vi "Frame.Settings.vi"(6 "Action":enum8{"Get", "Set"}(ring), 8 "error in (no error)":errorcluster, 10 "Frame.Settings":T1={"ID"=0, "Disable Transmission"=FALSE, "Disable Transmission Ref"=18446744073709551615, "Transmit Trigger"=enum."Channel value change", "Transmit Trigger Ref"=18446744073709551615, "Start Time Offset (ms)"=0} {"Transmit Trigger Ref" format="%.0x"; "Disable Transmission Ref" format="%.0x"}, 11 "Item Ref in":T2 format="%.0x") -> (0 "error out":errorcluster, 2 "Frame.Settings":T1={"ID"=0, "Disable Transmission"=FALSE, "Disable Transmission Ref"=18446744073709551615, "Transmit Trigger"=enum."Channel value change", "Transmit Trigger Ref"=18446744073709551615, "Start Time Offset (ms)"=0} {"Transmit Trigger Ref" format="%.0x"; "Disable Transmission Ref" format="%.0x"}, 3 "Item Ref out":T2 format="%.0x")   [LabVIEW 2023, in "Protection and Counter Addon System Explorer.lvlib"]
uses:
  Protection and Counter Addon System Explorer.lvlib
  <vilib>/NI VeriStand/Custom Device API/Custom Device Item Ref.ctl
  Types/Frame Settings.ctl
  Types/Event Trigger Type.ctl
  Addon Shared/SubVIs/GUID Lookup.vi
  <vilib>/NI VeriStand/Custom Device API/Set Item Property (Dependent Node Pointer).vi
  <vilib>/NI VeriStand/Custom Device API/Set Item Property (U32).vi
  <vilib>/NI VeriStand/Custom Device API/Set Item Property (Boolean).vi
  <vilib>/NI VeriStand/Custom Device API/Get Item Property (Dependent Node Pointer).vi
  <vilib>/NI VeriStand/Custom Device API/Get Item Property (U32).vi
  <vilib>/NI VeriStand/Custom Device API/Get Item Property (Boolean).vi
  <vilib>/NI VeriStand/Custom Device API/Custom Device API.lvlib
  Addon Shared/Protection and Counter Addon Shared.lvlib
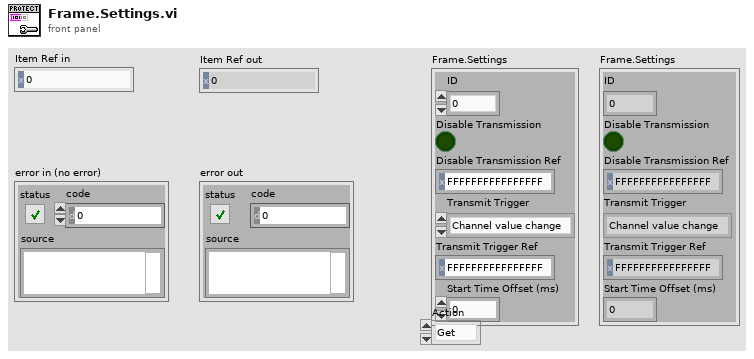
[diagram p1: front panel]
types:
  T1 = typedef "Protection and Counter Addon System Explorer.lvlib/Frame Settings.ctl" = cluster{"ID":u32, "Disable Transmission":bool, "Disable Transmission Ref":T2, "Transmit Trigger":T3, "Transmit Trigger Ref":T2, "Start Time Offset (ms)":u32}
  T2 = typedef "Custom Device API.lvlib/Custom Device Item Ref.ctl" = u64
  T3 = typedef "Protection and Counter Addon System Explorer.lvlib/Event Trigger Type.ctl" = enum16{"Channel value change", "Trigger channel (not zero)", "Channel value change or trigger channel (not zero)", "Trigger channel (any value change)", "Channel value change or trigger channel (any value change)"}
  T4 = typedef "Custom Device API.lvlib/Custom Device Item Info.ctl" = cluster{"Name":string, "Is Channel":bool, "GUID":string, "Is Waveform":bool}
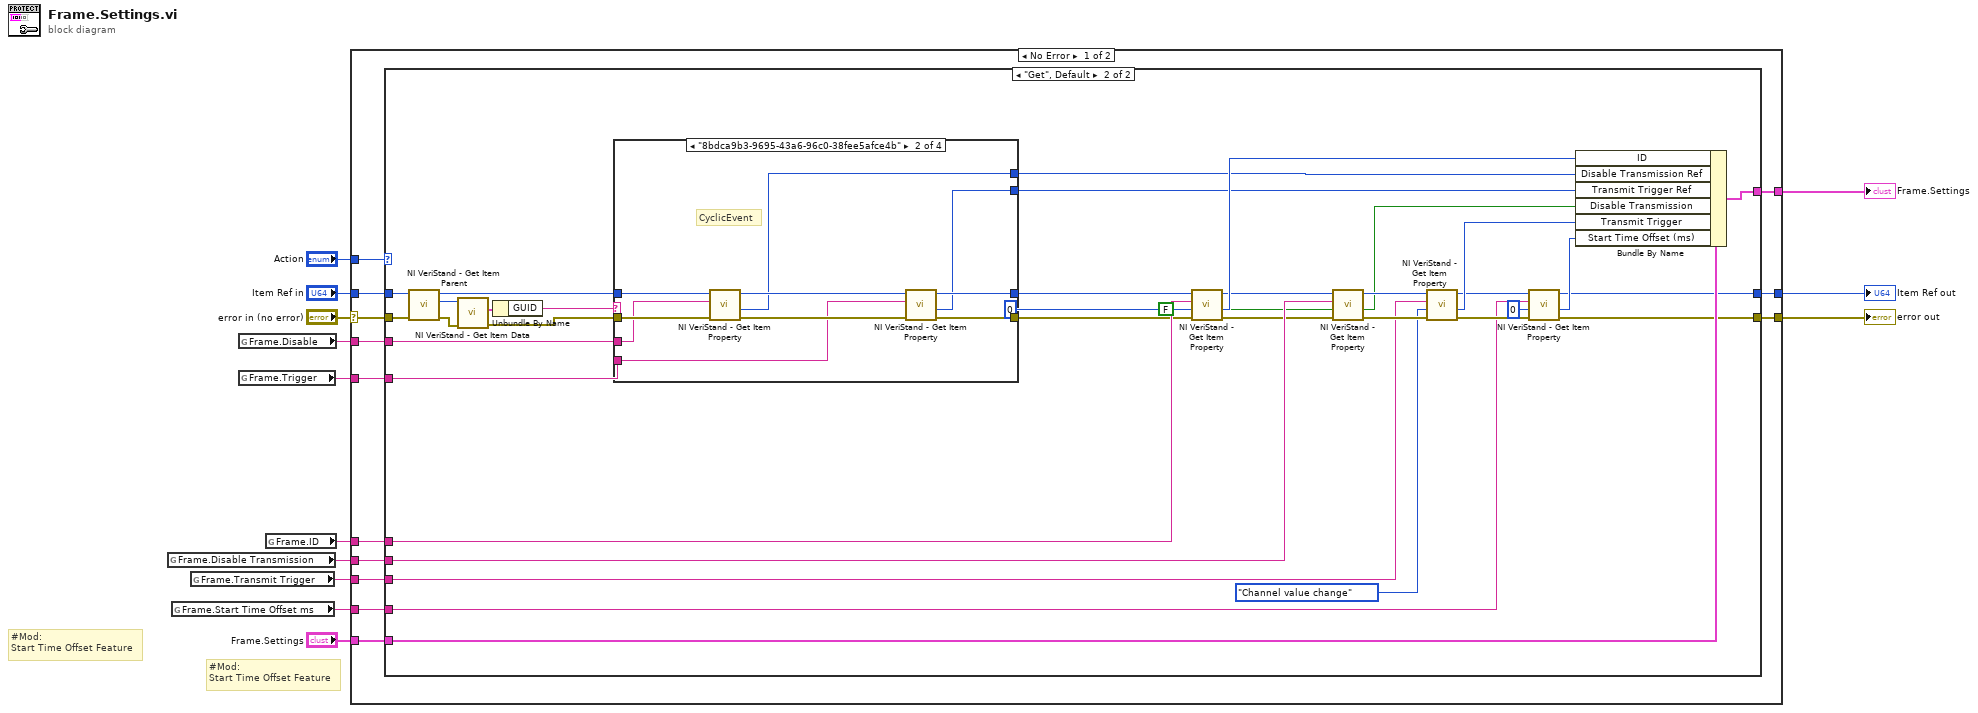
[diagram p0: block diagram]
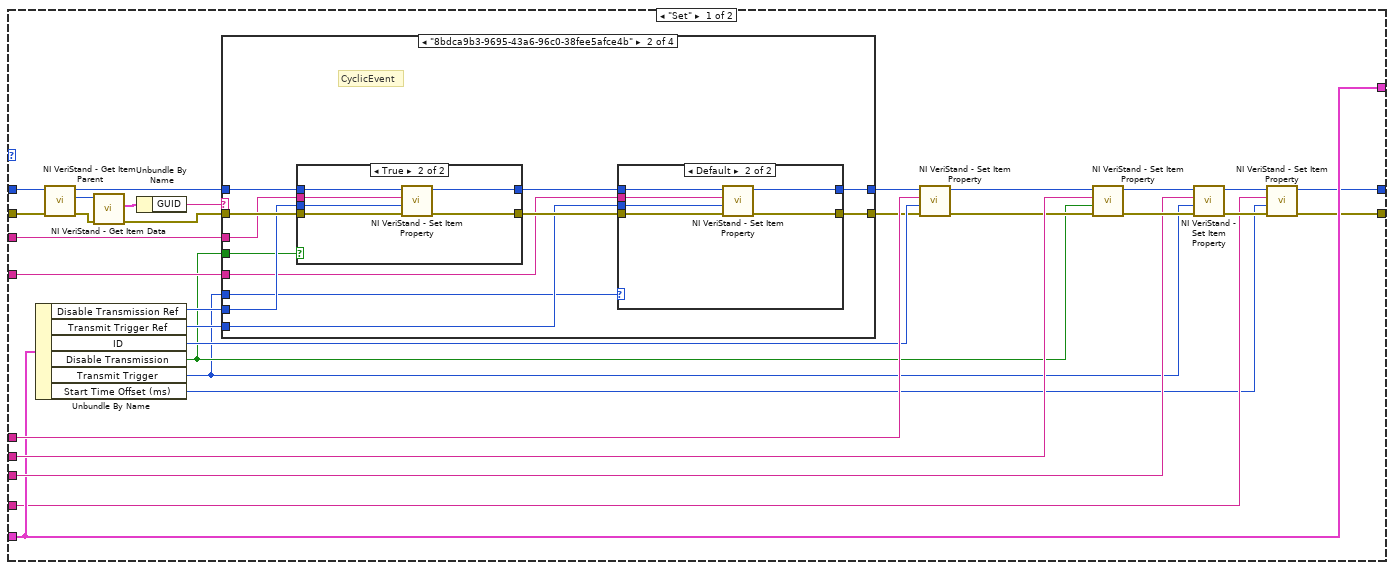
[diagram p2: hidden frame]
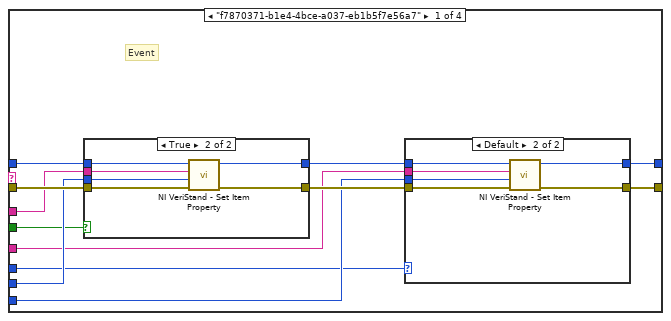
[diagram p3: hidden frame]
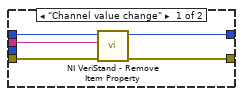
[diagram p4: hidden frame]
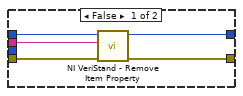
[diagram p5: hidden frame]
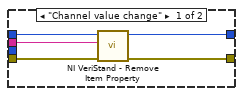
[diagram p6: hidden frame]
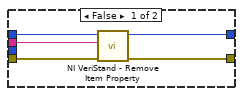
[diagram p7: hidden frame]
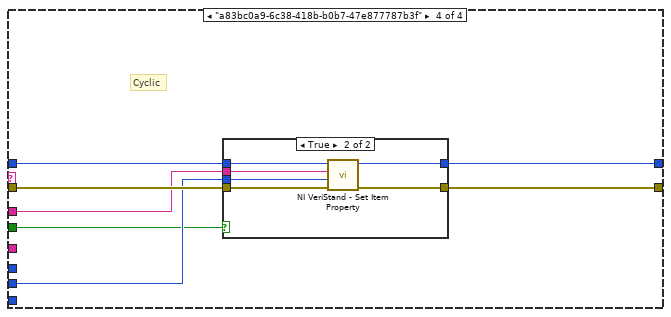
[diagram p9: hidden frame]
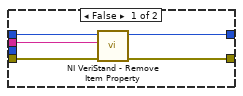
[diagram p10: hidden frame]
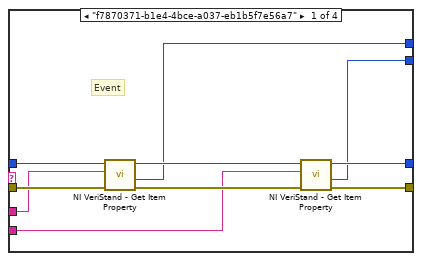
[diagram p11: hidden frame]
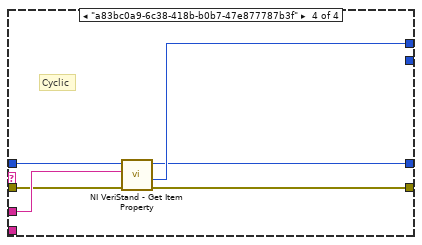
[diagram p13: hidden frame]
diagram:
  # "#Mod:\nStart Time Offset Feature"
  # "#Mod:\nStart Time Offset Feature"
  n1 = global read "GUID Lookup.vi" "Frame.Disable Transmission"() -> (w5:string)
  n2 = global read "GUID Lookup.vi" "Frame.Start Time Offset ms"() -> (w1:string)
  n3 = global read "GUID Lookup.vi" "Frame.Transmit Trigger"() -> (w6:string)
  n4 = global read "GUID Lookup.vi" "Frame.Disable"() -> (w2:string)
  n5 = global read "GUID Lookup.vi" "Frame.Trigger"() -> (w3:string)
  n6 = global read "GUID Lookup.vi" "Frame.ID"() -> (w4:string)
  n7 = case shown="No Error" "error in (no error)" {
    selector: "error in (no error)" -> [w17 w210]
    tunnel: "Item Ref in" -> [w26 w209]
    tunnel: w4 -> [w25 _]
    tunnel: w2 -> [w24 _]
    tunnel: w3 -> [w23 _]
    tunnel: [w22 w210] -> w12
    tunnel: [w21 w209] -> w11
    tunnel: [w20 _] -> w10
    tunnel: w6 -> [w19 _]
    tunnel: w5 -> [w18 _]
    tunnel: "Frame.Settings" -> [w16 _]
    tunnel: "Action" -> [w15 _]
    tunnel: w1 -> [w14 _]
    frame No Error {
      n8 = case shown="\"Get\", Default" w15 {
        tunnel: w26 -> [w45 w162]
        tunnel: w25 -> [w56 w180]
        tunnel: w24 -> [w42 w157]
        tunnel: w23 -> [w41 w156]
        tunnel: [w31 w145] -> w22
        tunnel: [w27 w146] -> w21
        tunnel: [w51 w170] -> w20
        tunnel: w19 -> [w53 w176]
        tunnel: w18 -> [w52 w175]
        tunnel: w17 -> [w44 w159]
        tunnel: w16 -> [w51 w171]
        tunnel: w14 -> [w29 w149]
        frame "Set" {
          n9 = Unbundle By Name(w51) -> ("Disable Transmission Ref"=w36:T2, "Transmit Trigger Ref"=w35:T2, "ID"=w50:u32, "Disable Transmission"=w34:bool, "Transmit Trigger"=w33:T3, "Start Time Offset (ms)"=w28:u32)
          n10 = call <vilib>:"NI VeriStand - Get Item Parent.vi"("error in (no error)"=w44, "Item Ref in"=w45) -> ("error out"=w40:errorcluster, "Parent Ref"=w47:T2, "Item Ref out"=w46:T2)  [unwired: 6 in, 1 out]
          n11 = call <vilib>:"NI VeriStand - Get Item Data.vi"("error in (no error)"=w40, "Item Ref in"=w47) -> ("error out"=w43:errorcluster, "Item Info"=w48:T4)  [unwired: 8 out]
          n12 = Unbundle By Name(w48) -> ("GUID"=w49:string)
          n13 = case shown="\"8bdca9b3-9695-43a6-96c0-38fee5afce4b\"" w49 {
            tunnel: w43 -> [w68 w102 w126 w133]
            tunnel: [w58 w92 w126 w128] -> w39
            tunnel: w42 -> [w67 w101 _ w131]
            tunnel: w41 -> [w61 w95 _ _]
            tunnel: w46 -> [w66 w100 w125 w130]
            tunnel: [w59 w93 w125 w129] -> _
            tunnel: w36 -> [w65 w99 _ w132]
            tunnel: w35 -> [w62 w96 _ _]
            tunnel: w34 -> [w64 w98 _ w127]
            tunnel: w33 -> [w57 w91 _ _]
            frame "f7870371-b1e4-4bce-a037-eb1b5f7e56a7" {
              # "Event"
              n14 = case shown="True" w64 {
                tunnel: [w80 w90] -> w60
                tunnel: [w81 w89] -> w63
                tunnel: w68 -> [w82 w88]
                tunnel: w67 -> [w83 w87]
                tunnel: w66 -> [w84 w86]
                tunnel: w65 -> [_ w85]
                frame False {
                  n15 = call <vilib>:"NI VeriStand - Remove Item Property.vi"("error in (no error)"=w82, "Property Name"=w83, "Item Ref in"=w84) -> ("error out"=w81:errorcluster, "Item Ref out"=w80:T2)  [unwired: 6 in, 1 out]
                }
                frame True {
                  n16 = call-poly <vilib>:"NI VeriStand - Set Item Property.vi"("error in (no error)"=w88, "Dependent Node Ref"=w85, "Property Name"=w87, "Item Ref in"=w86) -> ("error out"=w89:errorcluster, "Item Ref out"=w90:T2)  [unwired: 5 in, 1 out]
                }
              }
              n17 = case shown="Default" w57 {
                tunnel: [w69 w79] -> w59
                tunnel: [w70 w78] -> w58
                tunnel: w63 -> [w71 w77]
                tunnel: w61 -> [w72 w76]
                tunnel: w60 -> [w73 w75]
                tunnel: w62 -> [_ w74]
                frame "Channel value change" {
                  n18 = call <vilib>:"NI VeriStand - Remove Item Property.vi"("error in (no error)"=w71, "Property Name"=w72, "Item Ref in"=w73) -> ("error out"=w70:errorcluster, "Item Ref out"=w69:T2)  [unwired: 6 in, 1 out]
                }
                frame Default {
                  n19 = call-poly <vilib>:"NI VeriStand - Set Item Property.vi"("error in (no error)"=w77, "Dependent Node Ref"=w74, "Property Name"=w76, "Item Ref in"=w75) -> ("error out"=w78:errorcluster, "Item Ref out"=w79:T2)  [unwired: 5 in, 1 out]
                }
              }
            }
            frame "8bdca9b3-9695-43a6-96c0-38fee5afce4b" {
              # "CyclicEvent"
              n20 = case shown="True" w98 {
                tunnel: [w114 w124] -> w94
                tunnel: [w115 w123] -> w97
                tunnel: w102 -> [w116 w122]
                tunnel: w101 -> [w117 w121]
                tunnel: w100 -> [w118 w120]
                tunnel: w99 -> [_ w119]
                frame False {
                  n21 = call <vilib>:"NI VeriStand - Remove Item Property.vi"("error in (no error)"=w116, "Property Name"=w117, "Item Ref in"=w118) -> ("error out"=w115:errorcluster, "Item Ref out"=w114:T2)  [unwired: 6 in, 1 out]
                }
                frame True {
                  n22 = call-poly <vilib>:"NI VeriStand - Set Item Property.vi"("error in (no error)"=w122, "Dependent Node Ref"=w119, "Property Name"=w121, "Item Ref in"=w120) -> ("error out"=w123:errorcluster, "Item Ref out"=w124:T2)  [unwired: 5 in, 1 out]
                }
              }
              n23 = case shown="Default" w91 {
                tunnel: [w103 w113] -> w93
                tunnel: [w104 w112] -> w92
                tunnel: w97 -> [w105 w111]
                tunnel: w95 -> [w106 w110]
                tunnel: w94 -> [w107 w109]
                tunnel: w96 -> [_ w108]
                frame "Channel value change" {
                  n24 = call <vilib>:"NI VeriStand - Remove Item Property.vi"("error in (no error)"=w105, "Property Name"=w106, "Item Ref in"=w107) -> ("error out"=w104:errorcluster, "Item Ref out"=w103:T2)  [unwired: 6 in, 1 out]
                }
                frame Default {
                  n25 = call-poly <vilib>:"NI VeriStand - Set Item Property.vi"("error in (no error)"=w111, "Dependent Node Ref"=w108, "Property Name"=w110, "Item Ref in"=w109) -> ("error out"=w112:errorcluster, "Item Ref out"=w113:T2)  [unwired: 5 in, 1 out]
                }
              }
            }
            frame "45d997b9-be87-4536-8aa7-486032a53b20", Default {
              # "SinglePoint"
            }
            frame "a83bc0a9-6c38-418b-b0b7-47e877787b3f" {
              # "Cyclic"
              n26 = case shown="True" w127 {
                tunnel: [w134 w144] -> w129
                tunnel: [w135 w143] -> w128
                tunnel: w133 -> [w136 w142]
                tunnel: w131 -> [w137 w141]
                tunnel: w130 -> [w138 w140]
                tunnel: w132 -> [_ w139]
                frame False {
                  n27 = call <vilib>:"NI VeriStand - Remove Item Property.vi"("error in (no error)"=w136, "Property Name"=w137, "Item Ref in"=w138) -> ("error out"=w135:errorcluster, "Item Ref out"=w134:T2)  [unwired: 6 in, 1 out]
                }
                frame True {
                  n28 = call-poly <vilib>:"NI VeriStand - Set Item Property.vi"("error in (no error)"=w142, "Dependent Node Ref"=w139, "Property Name"=w141, "Item Ref in"=w140) -> ("error out"=w143:errorcluster, "Item Ref out"=w144:T2)  [unwired: 5 in, 1 out]
                }
              }
            }
          }
          n29 = call-poly <vilib>:"NI VeriStand - Set Item Property.vi"("error in (no error)"=w39, "Value"=w50, "Property Name"=w56, "Item Ref in"=w45) -> ("error out"=w38:errorcluster, "Item Ref out"=w37:T2)  [unwired: 5 in, 1 out]
          n30 = call-poly <vilib>:"NI VeriStand - Set Item Property.vi"("error in (no error)"=w38, "Value"=w34, "Property Name"=w52, "Item Ref in"=w37) -> ("error out"=w54:errorcluster, "Item Ref out"=w55:T2)  [unwired: 5 in, 1 out]
          n31 = call-poly <vilib>:"NI VeriStand - Set Item Property.vi"("error in (no error)"=w54, "Value"=w33, "Property Name"=w53, "Item Ref in"=w55) -> ("error out"=w32:errorcluster, "Item Ref out"=w30:T2)  [unwired: 5 in, 1 out]
          n32 = call-poly <vilib>:"NI VeriStand - Set Item Property.vi"("error in (no error)"=w32, "Value"=w28, "Property Name"=w29, "Item Ref in"=w30) -> ("error out"=w31:errorcluster, "Item Ref out"=w27:T2)  [unwired: 5 in, 1 out]
        }
        frame "Get", Default {
          n33 = call <vilib>:"NI VeriStand - Get Item Parent.vi"("error in (no error)"=w159, "Item Ref in"=w162) -> ("error out"=w163:errorcluster, "Parent Ref"=w164:T2, "Item Ref out"=w155:T2)  [unwired: 6 in, 1 out]
          n34 = call <vilib>:"NI VeriStand - Get Item Data.vi"("error in (no error)"=w163, "Item Ref in"=w164) -> ("error out"=w165:errorcluster, "Item Info"=w166:T4)  [unwired: 8 out]
          n35 = Unbundle By Name(w166) -> ("GUID"=w167:string)
          n36 = case shown="\"8bdca9b3-9695-43a6-96c0-38fee5afce4b\"" w167 {
            tunnel: w165 -> [w188 w198 w202 w206]
            tunnel: [w187 w197 w202 w205] -> w158
            tunnel: w157 -> [w186 w196 _ w208]
            tunnel: w156 -> [w185 w195 _ _]
            tunnel: w155 -> [w184 w194 w201 w207]
            tunnel: [w183 w193 w201 w203] -> w154
            tunnel: [w182 w192 _ w204] -> w153
            tunnel: [w181 w191 _ _] -> w152
            frame "f7870371-b1e4-4bce-a037-eb1b5f7e56a7" {
              # "Event"
              n37 = call-poly <vilib>:"NI VeriStand - Get Item Property.vi"("error in (no error)"=w188, "Property Name"=w186, "Item Ref in"=w184) -> ("error out"=w189:errorcluster, "Dependent Node Ref"=w182:T2, "Item Ref out"=w190:T2)  [unwired: 5 in, 1 out]
              n38 = call-poly <vilib>:"NI VeriStand - Get Item Property.vi"("error in (no error)"=w189, "Property Name"=w185, "Item Ref in"=w190) -> ("error out"=w187:errorcluster, "Dependent Node Ref"=w181:T2, "Item Ref out"=w183:T2)  [unwired: 5 in, 1 out]
            }
            frame "8bdca9b3-9695-43a6-96c0-38fee5afce4b" {
              # "CyclicEvent"
              n39 = call-poly <vilib>:"NI VeriStand - Get Item Property.vi"("error in (no error)"=w198, "Property Name"=w196, "Item Ref in"=w194) -> ("error out"=w199:errorcluster, "Dependent Node Ref"=w192:T2, "Item Ref out"=w200:T2)  [unwired: 5 in, 1 out]
              n40 = call-poly <vilib>:"NI VeriStand - Get Item Property.vi"("error in (no error)"=w199, "Property Name"=w195, "Item Ref in"=w200) -> ("error out"=w197:errorcluster, "Dependent Node Ref"=w191:T2, "Item Ref out"=w193:T2)  [unwired: 5 in, 1 out]
            }
            frame "45d997b9-be87-4536-8aa7-486032a53b20", Default {
              # "SinglePoint"
            }
            frame "a83bc0a9-6c38-418b-b0b7-47e877787b3f" {
              # "Cyclic"
              n41 = call-poly <vilib>:"NI VeriStand - Get Item Property.vi"("error in (no error)"=w206, "Property Name"=w208, "Item Ref in"=w207) -> ("error out"=w205:errorcluster, "Dependent Node Ref"=w204:T2, "Item Ref out"=w203:T2)  [unwired: 5 in, 1 out]
            }
          }
          n42 = call-poly <vilib>:"NI VeriStand - Get Item Property.vi"("error in (no error)"=w158, "Default Value"=u32 0, "Property Name"=w180, "Item Ref in"=w154) -> ("error out"=w161:errorcluster, "Value"=w174:u32, "Item Ref out"=w160:T2)  [unwired: 4 in, 1 out]
          n43 = call-poly <vilib>:"NI VeriStand - Get Item Property.vi"("error in (no error)"=w161, "Default Value"=FALSE, "Property Name"=w175, "Item Ref in"=w160) -> ("error out"=w177:errorcluster, "Value"=w172:bool, "Item Ref out"=w178:T2)  [unwired: 4 in, 1 out]
          n44 = call-poly <vilib>:"NI VeriStand - Get Item Property.vi"("error in (no error)"=w177, "Default Value"=Event_Trigger_Type."Channel value change" ("Transmit Trigger"), "Property Name"=w176, "Item Ref in"=w178) -> ("error out"=w150:errorcluster, "Value"=w173:u32, "Item Ref out"=w151:T2)  [unwired: 4 in, 1 out]
          n45 = call-poly <vilib>:"NI VeriStand - Get Item Property.vi"("error in (no error)"=w150, "Default Value"=u32 0, "Property Name"=w149, "Item Ref in"=w151) -> ("error out"=w145:errorcluster, "Value"=w147:u32, "Item Ref out"=w146:T2)  [unwired: 4 in, 1 out]
          n46 = Bundle By Name(cluster=w171, "ID"=w174, "Disable Transmission Ref"=w153, "Transmit Trigger Ref"=w152, "Disable Transmission"=w172, "Transmit Trigger"=w173, "Start Time Offset (ms)"=w147) -> (w170:T1)
        }
      }
    }
    frame Error {
    }
  }
  "Item Ref out" <- w11
  "error out" <- w12
  "Frame.Settings" <- w10
